vi "CRYAPI Get Boolean Reference.vi"(8 "Label Name":string, 11 "VI Refnum":refnum<vi>) -> (1 "Boolean":bool, 2 "Boolean Ref":refnum<vi>, 3 "VI Refnum Out":refnum<vi>)   [LabVIEW 2013]
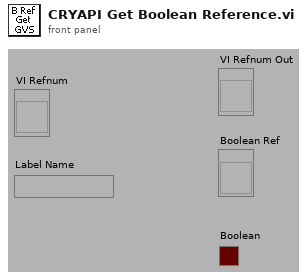
[diagram p1: front panel]
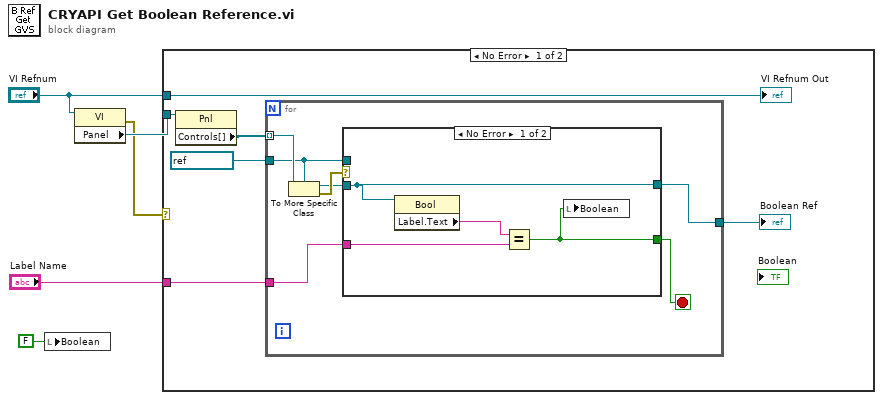
[diagram p0: block diagram]
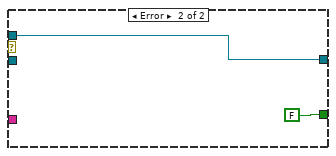
[diagram p2: hidden frame]
diagram:
  n1 = local write "Boolean"(FALSE ("Boolean")) -> ()
  n2 = property class="VI"(reference="VI Refnum") -> (error out=w1:errorcluster, "Panel"=w3:refnum<vi>)  [unwired: 1 in, 1 out]
  n3 = case shown="No Error" w1 {
    tunnel: "Label Name" -> [w11 _]
    tunnel: w3 -> [w10 _]
    tunnel: "VI Refnum" -> [w8 _]
    frame No Error {
      n4 = property class="Pnl"(reference=w10) -> ("Controls[]"=w9:refnum<vi>[])  [unwired: 1 in, 2 out]
      n5 = for {
        tunnel: w9 -> [w18] mode=indexing
        tunnel: [w14] -> w7
        tunnel: w11 -> [w13]
        tunnel: refnum<vi> refnum ("Boolean") -> [w12]
        stop <- w15 stop-if-true
        n6 = To More Specific Class(target class=w12, reference=w18) -> (specific class reference=w16:refnum<vi>, error out=w17:errorcluster)  [unwired: 1 in]
        n7 = case shown="No Error" w17 {
          tunnel: w16 -> [w20 _]
          tunnel: [w19 FALSE] -> w15
          tunnel: [w20 w23] -> w14
          tunnel: w13 -> [w21 _]
          tunnel: w12 -> [_ w23]
          frame No Error {
            n8 = property class="Bool"(reference=w20) -> ("Label.Text"=w22:string)  [unwired: 1 in, 2 out]
            n9 = Equal?(x=w22, y=w21) -> (x = y?=w19:bool)
            n10 = local write "Boolean"(w19) -> ()
          }
          frame Error {
          }
        }
      }
      "Boolean Ref" <- w7
      "VI Refnum Out" <- w8
    }
    frame Error {
    }
  }
